vi "Arithmetic Shift.vi"(1 "x":i16 format="%016b", 2 "y":i16 format="%016b") -> (0 "x << y":i16 format="%016b")   [LabVIEW 2020, in "Protobuf RAW.lvlib"]
uses:
  Protobuf RAW.lvlib
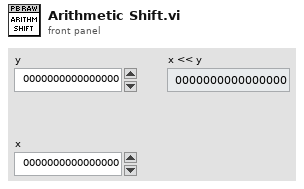
[diagram p1: front panel]
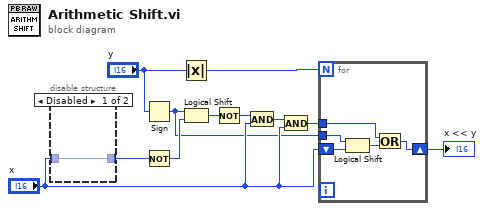
[diagram p0: block diagram]
diagram:
  n1 = disable-structure shown="Disabled" {
    disable-tunnel: [w12 _] -> w11
    disable-tunnel: "x" -> [w12 _]
    frame Disabled {
    }
    frame Enabled {
    }
  }
  n2 = Sign(1:"y") -> (0:w2:i16)
  n3 = Not(x=w11) -> (.not. x?=w7:i16)
  n4 = Absolute Value(x="y") -> (abs(x)=w1:i16)
  n5 = Logical Shift(y=w2, x=w7) -> (x << y=w4:i16)
  n6 = Not(x=w4) -> (.not. x?=w3:i16)
  n7 = And(x=w3, y="x") -> (x .and. y?=w5:i16)
  n8 = And(x=w5, y="x") -> (x .and. y?=w10:i16)
  n9 = for {
    N: w1 -> [_]
    tunnel: w10 -> [w16]
    tunnel: w2 -> [w13]
    shift-right: [w15] -> w9
    shift-left: "x" -> [w14]
    n10 = Logical Shift(y=w13, x=w14) -> (x << y=w17:i16)
    n11 = Or(x=w16, y=w17) -> (x .or. y?=w15:i16)
  }
  "x << y" <- w9
